vi "Element Init.vi"(7 "VolatusAPI":refnum<class "VolatusAPI.lvclass">, 8 "error in (no error)":errorcluster, 10 "JSON":string, 11 "BooleanControl in":refnum<class "BooleanControl.lvclass">) -> (0 "error out":errorcluster, 3 "BooleanControl out":refnum<class "BooleanControl.lvclass">)   [LabVIEW 2020, in "VolatusGUIElements.lvlib" / "BooleanControl.lvclass"]
uses:
  BooleanControl.lvclass
  C:/dev/lv20CE/relink/lv-volatus/VolatusGUI/GUI Element/GUI Element.lvclass
  Volatus/VolatusAPI/VolatusAPI.lvclass
  JSON.ctl
  lv-vecto/Vecto/Group DBL/Group DBL.lvclass
  C:/dev/lv20CE/relink/lv-vecto/Vecto/Group/Group.lvclass
  VolatusGUI/GUI Element/GUI Element.lvclass/GUI Element.ctl
  BooleanControl.lvclass/BooleanControl.ctl
  34537da6-9836-4c71-8cf0-a3fcb64d615c.vi
  <vilib>/JDP Science/JSONtext/JSON text to Variant.vi
  <vilib>/JDP Science/JSONtext/LVClass Serializer/JSONtext LVClass Serializer.lvclass
  VolatusGUI/GUI Element/GUI Element.lvclass
  VolatusGUI/Element Inhibit/Element Inhibit.lvclass
  Volatus/Digital Command/Digital Command.lvclass
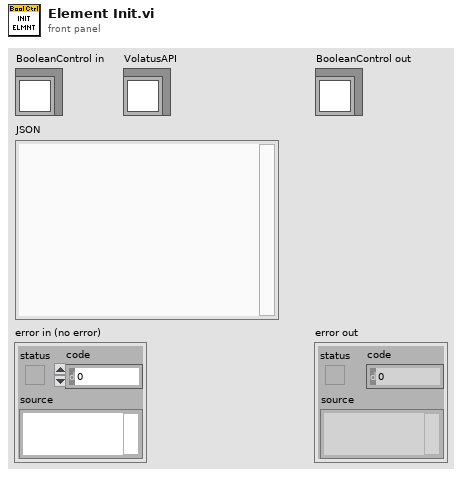
[diagram p1: front panel]
types:
  T1 = typedef "VolatusGUIElements.lvlib/BooleanControl.lvclass/JSON.ctl" = cluster{"Channel":string, "Inhibit":string}
  T2 = typedef "VectoConfig.lvlib/Channel Info.ctl" = cluster{"Name":string, "Group":string, "Owning Node":string, "Owning Task":string, "Resource":string}
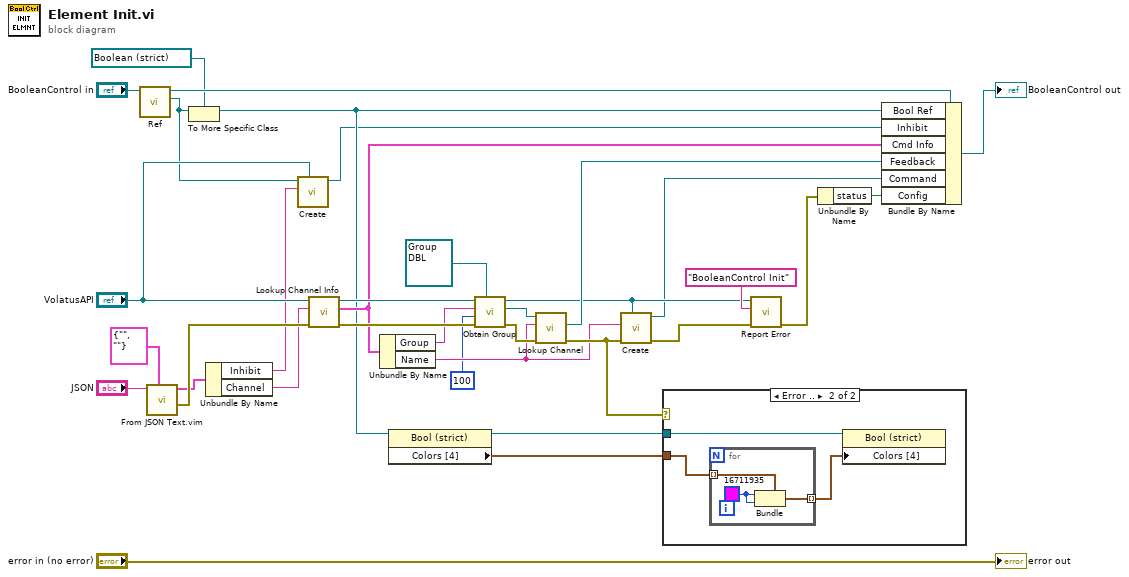
[diagram p0: block diagram]
diagram:
  n1 = call "Ref.vi"("GUI Element in"="BooleanControl in") -> ("Ref"=w9:refnum<vi>, "GUI Element out"=w29:refnum<class "BooleanControl.lvclass">)  [unwired: 9 in]
  n2 = call "From JSON Text.vim"("Data Type and Default Value"=T1 {"Channel"="", "Inhibit"=""} ("JSON"), "JSON"="JSON") -> ("error out"=w34:errorcluster, "Data out"=w26:T1)  [unwired: 8 in]
  n3 = To More Specific Class(target class=refnum<vi> refnum ("Auto Spark"), reference=w9) -> (specific class reference=w14:refnum<vi>)  [unwired: 1 in, 1 out]
  n4 = Unbundle By Name(w26) -> ("Inhibit"=w10:string, "Channel"=w19:string)
  n5 = call "Create.vi"("VolatusAPI"="VolatusAPI", "Inhibit Channel"=w10, "Control Ref"=w9) -> ("Element Inhibit out"=w8:refnum<class "Element Inhibit.lvclass">)  [unwired: 7 in, 1 out]
  n6 = call "Lookup Channel Info.vi"("error in (no error)"=w34, "Channel Name"=w19, "VolatusAPI in"="VolatusAPI") -> ("error out"=w22:errorcluster, "Channel Info"=w18:T2, "VolatusAPI out"=w21:refnum<class "VolatusAPI.lvclass">)  [unwired: 5 in, 1 out]
  n7 = Unbundle By Name(w18) -> ("Group"=w20:string, "Name"=w5:string)
  n8 = property class="Bool (strict)"(reference=w14) -> (reference out=w13:refnum<vi>, "Colors [4]"=w15:cluster{u32, u32}[])  [unwired: 1 in, 1 out]
  n9 = call "Obtain Group.vi"("Group Type (Abstract)"=refnum<class "Group DBL.lvclass"> refnum ("Vecto.lvlib:Group.lvclass"), "error in (no error)"=w22, "Timeout ms (5000)"=u32 100, "Group Name"=w20, "VolatusAPI in"=w21) -> ("error out"=w23:errorcluster, "Group"=w24:refnum<class "Group DBL.lvclass">, "VolatusAPI out"=w4:refnum<class "VolatusAPI.lvclass">)  [unwired: 4 in]
  n10 = call "Lookup Channel.vi"("error in (no error)"=w23, "Channel Name"=w5, "Group in"=w24) -> ("error out"=w7:errorcluster, "Channel"=w17:refnum<class "Channel DBL.lvclass">)  [unwired: 6 in, 1 out]
  n11 = call "Create.vi"("VolatusAPI"=w4, "error in (no error)"=w7, "Channel"=w5) -> ("error out"=w2:errorcluster, "Digital Command out"=w3:refnum<class "Digital Command.lvclass">)  [unwired: 7 in]
  n12 = case shown="Error .." w7 {
    tunnel: w15 -> [_ w36]
    tunnel: w13 -> [_ w37]
    frame No Error {
    }
    frame Error {
      n13 = for {
        tunnel: w36 -> [w40] mode=indexing
        tunnel: [w39] -> w35 mode=indexing
        w38 = u32 16711935
        n14 = Bundle(cluster=w40, w38, w38) -> (w39:cluster{u32, u32})
      }
      n15 = property class="Bool (strict)"(reference=w37, "Colors [4]"=w35) -> ()  [unwired: 1 in, 2 out]
    }
  }
  n16 = call "Report Error.vi"("error in (no error)"=w2, "Context"="BooleanControl Init", "VolatusAPI in"=w4) -> ("error out"=w6:errorcluster)  [unwired: 7 in, 1 out]
  n17 = Unbundle By Name(w6) -> ("status"=w12:bool)
  n18 = Bundle By Name(cluster=w29, "Bool Ref"=w14, "Inhibit"=w8, "Cmd Info"=w18, "Feedback"=w17, "Command"=w3, "Config"=w12) -> (→"BooleanControl out":refnum<class "BooleanControl.lvclass">)
  "error out" <- "error in (no error)"
